vi "Initialize.vi"(8 "error in (no error)":errorcluster, 11 "MDPtrMgr in":refnum<class "MDPtrMgr.lvclass">) -> (0 "error out":errorcluster, 3 "MDPtrMgr out":refnum<class "MDPtrMgr.lvclass">)   [LabVIEW 2017, in "MDPtr.lvlib" / "MDPtrMgr.lvclass"]
uses:
  MDPtrMgr.lvclass
  MDPtrMgr.lvclass/MDPtrMgr.ctl
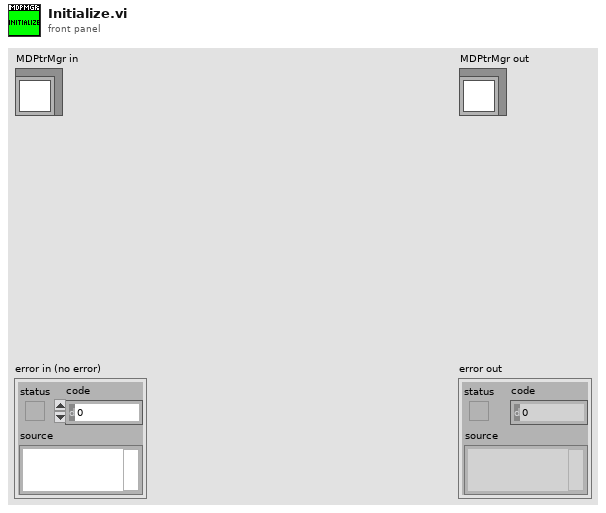
[diagram p1: front panel]
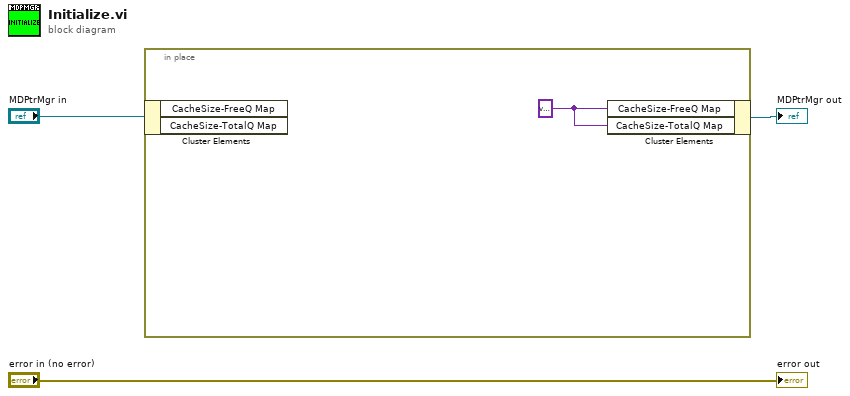
[diagram p0: block diagram]
diagram:
  n1 = in-place {
    w4 = variant ("FreeQueue")
    n2 = in-place-cluster #1("MDPtrMgr in") -> ()  [unwired: 2 out]
    n3 = in-place-cluster #1("CacheSize-FreeQ Map"=w4, "CacheSize-TotalQ Map"=w4) -> (→"MDPtrMgr out":refnum<class "MDPtrMgr.lvclass">)
  }
  "error out" <- "error in (no error)"
